vi "Unary UnaryTemplate.vi"(6 "contextId":T1, 8 "error in":errorcluster, 9 "timeout (ms)":i32=-1, 10 "Request Data":cluster{"Numeric":dbl}, 11 "gRPC ID":T1) -> (0 "error out":errorcluster, 2 "Response Data":cluster{"Numeric":dbl}, 3 "gRPC ID out":T1)   [LabVIEW 2024, in "Client Template.lvlib"]
uses:
  Client Template.lvlib
  gRPC lv Support/grpc-lvsupport/grpcId.ctl
  14406a1e-a7cf-4c24-99dd-691dd951f022.vi
  14035477-4c25-4107-8ed5-d0c4ef420ce5.vi
  bfa98ae1-a568-404c-8efc-8dad1b643b91.vi
  gRPC lv Support/grpc-lvsupport/TranslateGrpcError.vi
  gRPC lv Support/grpc-lvsupport/Create Occurance.vi
  <vilib>/Utility/error.llb/Error Cluster From Error Code.vi
  gRPC lv Support/grpc-lvsupport/Wait On Occurrence.vi
  gRPC lv Support/grpc-lvsupport/grpc-lvsupport.lvlib
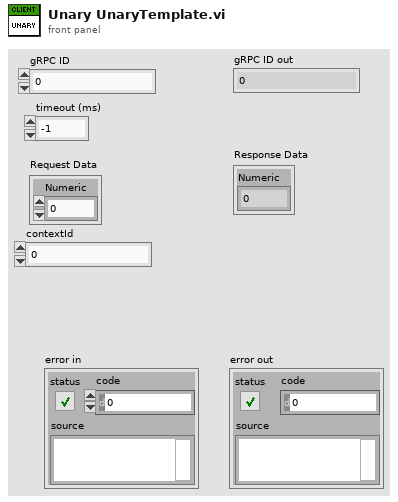
[diagram p1: front panel]
types:
  T1 = typedef "grpc-lvsupport.lvlib/grpcId.ctl" = u64
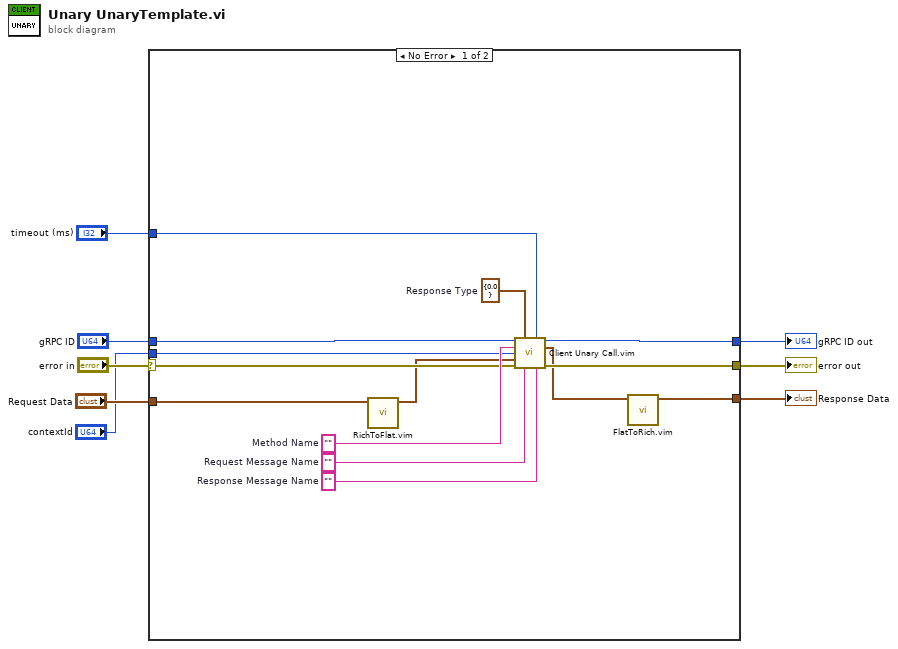
[diagram p0: block diagram]
diagram:
  n1 = case shown="No Error" "error in" {
    selector: "error in" -> [w18 w23]
    tunnel: [w17 w23] -> w7
    tunnel: "gRPC ID" -> [w16 w24]
    tunnel: [w15 w24] -> w5
    tunnel: "Request Data" -> [w12 _]
    tunnel: [w9 _] -> w3
    tunnel: "timeout (ms)" -> [w14 _]
    tunnel: "contextId" -> [w13 _]
    frame No Error {
      w19 = ""  # Response Message Name
      w20 = ""  # Request Message Name
      w21 = cluster{"Numeric":dbl} {"Numeric"=0.0}  # Response Type
      w22 = ""  # Method Name
      n2 = call "RichToFlat.vim"("InputCluster"=w12) -> ("OutputCluster"=w11:cluster{"Numeric":dbl})  [unwired: 10 in]
      n3 = call "Client Unary Call.vim"("ClientID in"=w16, "Response Type"=w21, "timeout (ms)"=w14, "Method Name"=w22, "contextId"=w13, "Request Data"=w11, "error in"=w18, "Request Message Name"=w20, "Response Message Name"=w19) -> ("ClientID out"=w15:u64, "Response Data"=w10:cluster{"Numeric":dbl}, "error out"=w17:errorcluster)  [unwired: 4 in]
      n4 = call "FlatToRich.vim"("InputCluster"=w10) -> ("OutputCluster"=w9:cluster{"Numeric":dbl})  [unwired: 10 in]
    }
    frame Error {
    }
  }
  "error out" <- w7
  "gRPC ID out" <- w5
  "Response Data" <- w3
